vi "Wave-Skip Chunk.vi"(8 "error in (no error)":errorcluster, 9 "Total bytes":u32, 10 "Bytes read":u32, 11 "refnum":refnum<file>) -> (0 "error out":errorcluster, 3 "refnum out":refnum<file>)   [LabVIEW 2020]
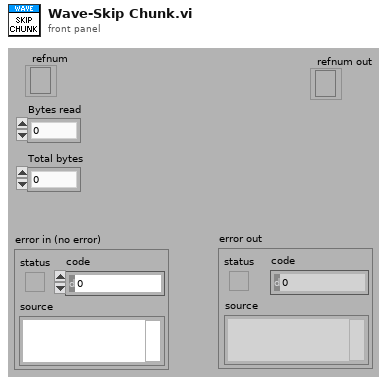
[diagram p1: front panel]
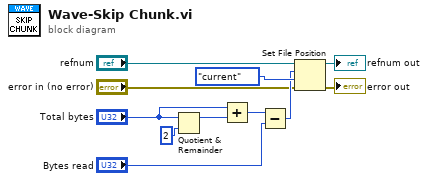
[diagram p0: block diagram]
diagram:
  n1 = Quotient & Remainder(x="Total bytes", y=2) -> (x-y*floor(x/y)=w11:u32)  [unwired: 1 out]
  n2 = Add(x="Total bytes", y=w11) -> (x+y=w2:u32)
  n3 = Subtract(x=w2, y="Bytes read") -> (x-y=w9:u32)
  n4 = Set File Position(offset (in bytes) (0)=w9, refnum="refnum", from (0:start)=enum16{"start", "end", "current"}."current", error in="error in (no error)") -> (refnum out=→"refnum out":refnum<file>, error out=→"error out":errorcluster)
